vi "Forward Message.vi"(6 "priority":i32, 8 "error in (no error)":errorcluster, 9 "Message in":refnum<class "Message.lvclass">, 10 "Target Enq":refnum<class "Message Enqueuer.lvclass">, 11 "Network Stream Writer in":refnum<class "Network Stream Writer.lvclass">) -> (0 "error out":errorcluster, 3 "Network Stream Writer out":refnum<class "Network Stream Writer.lvclass">)   [LabVIEW 2014, in "Network Stream Writer.lvlib" / "Network Stream Writer.lvclass"]
uses:
  Network Stream Writer.lvclass
  <vilib>/ActorFramework/Message/Message.lvclass
  <vilib>/ActorFramework/Message Enqueuer/Message Enqueuer.lvclass
  Network Stream/Network Stream/Network Stream.lvclass/Network Stream.ctl
  Proxy/Proxy/Proxy.lvclass/Proxy.ctl
  Network Stream Writer.lvclass/Network Stream Writer.ctl
  <vilib>/ActorFramework/Message Enqueuer/Message Priority.ctl
  Proxy/Proxy Messages/Return undeliverable Msg/Return undeliverable Msg.lvclass/Return undeliverable Msg.ctl
  <vilib>/ActorFramework/Message Enqueuer/Message Enqueuer.lvclass/Message Enqueuer.ctl
  <vilib>/ActorFramework/Message Enqueuer/Enqueue.vi
  <vilib>/ActorFramework/Message Priority Queue/Priority Enqueue.vi
  Proxy/Proxy Messages/Return undeliverable Msg/Return undeliverable Msg.lvclass
  Network Stream/Network Stream/Network Stream.lvclass
  Proxy/Proxy/Proxy.lvclass
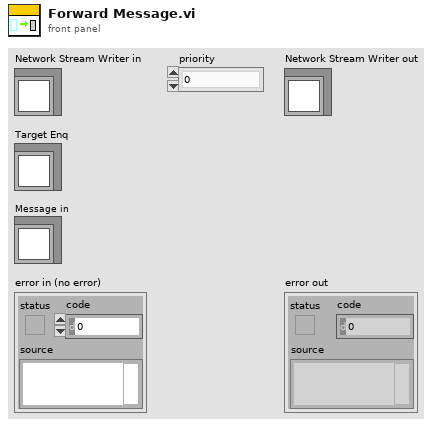
[diagram p1: front panel]
types:
  T1 = typedef "Network Stream.lvlib/Network Stream.lvclass/MessageString.ctl" = cluster{"Flatten Msg":string, "Message Priority":T2}
  T2 = typedef "Actor Framework.lvlib/Message Enqueuer.lvclass/Message Priority.ctl" = enum16{"Low", "Normal", "High"}
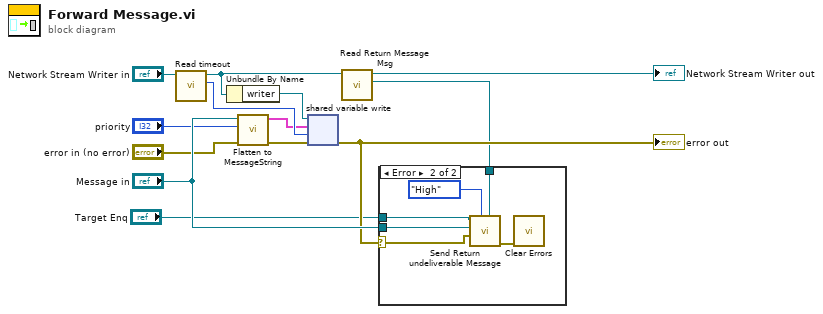
[diagram p0: block diagram]
diagram:
  n1 = call "Read timeout.vi"("Network Stream in"="Network Stream Writer in") -> ("timeout"=w10:i32, "Network Stream out"=w2:refnum<class "Network Stream Writer.lvclass">)  [unwired: 8 in, 1 out]
  n2 = Unbundle By Name(w2) -> ("writer"=w12:refnum<k21>)
  n3 = call "Flatten to MessageString.vi"("error in (no error)"="error in (no error)", "Message Priority"="priority", "Actor Framework:Message"="Message in") -> ("error out"=w6:errorcluster, "Msg String"=w8:T1)  [unwired: 7 in]
  n4 = shared-variable-write(w12, w6, w8, w10) -> (w5:errorcluster)  [unwired: 2 out]
  "error out" <- w5
  n5 = call "Read Return Message Msg.vi"("Proxy in"=w2) -> ("Proxy.lvlib:Return undeliverable Msg.lvclass"=w1:refnum<class "Return undeliverable Msg.lvclass">, "Proxy out"=→"Network Stream Writer out":refnum<class "Network Stream Writer.lvclass">)  [unwired: 8 in, 1 out]
  n6 = case shown="Error" w5 {
    selector: w5 -> [_ w18]
    tunnel: "Target Enq" -> [_ w19]
    tunnel: "Message in" -> [_ w17]
    tunnel: w1 -> [_ w14]
    frame No Error {
    }
    frame Error {
      n7 = call "Send Return undeliverable Message.vi"("Return Msg"=w14, "Message Priority (Normal)"=Message_Priority."High", "Tx Error"=w18, "Tx Message"=w17, "Message Enqueuer"=w19) -> ("error out"=w15:errorcluster)  [unwired: 5 in, 1 out]
      n8 = call <vilib>:"Clear Errors.vi"("error in (no error)"=w15) -> ()  [unwired: 5 in, 2 out]
    }
  }
